vi "Get Path List.vi"(5 "Drivers List":string[](array[string])) -> (4 "APIs Path":path[](array[path]))   [LabVIEW 2021, in "Path Functions.lvlib"]
uses:
  Path Functions.lvlib
  9bdd7397-0e0a-4018-8273-7dcc82681c82.vi
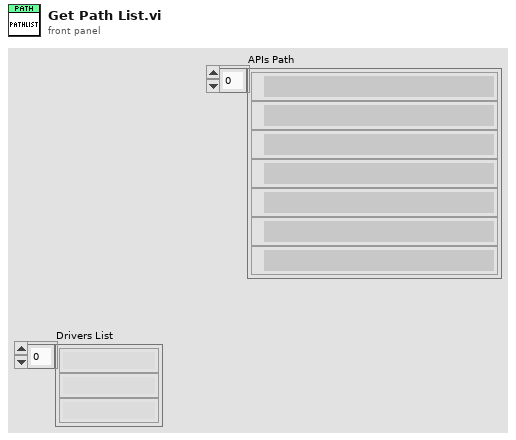
[diagram p1: front panel]
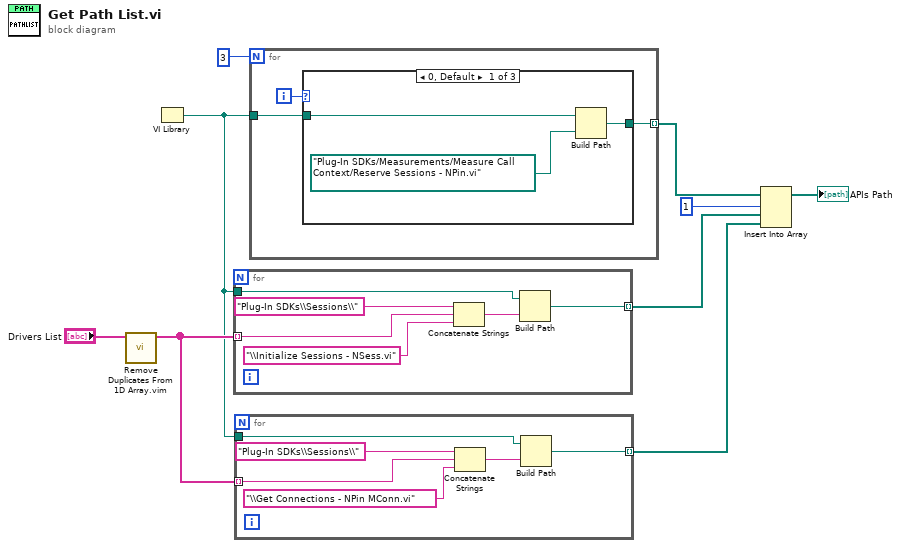
[diagram p0: block diagram]
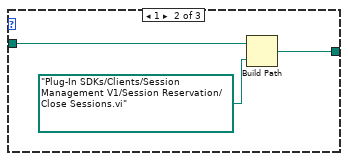
[diagram p2: hidden frame]
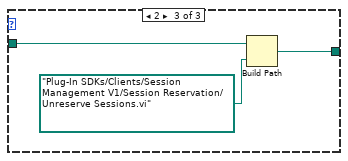
[diagram p3: hidden frame]
diagram:
  n1 = call "Remove Duplicates From 1D Array.vim"("array"="Drivers List") -> ("array with duplicates removed"=w2:string[])  [unwired: 10 in]
  n2 = VI Library() -> (path=w1:path)
  n3 = for {
    tunnel: w2 -> [w13] mode=indexing
    tunnel: w1 -> [w15]
    tunnel: [w10] -> w5 mode=indexing
    n4 = Concatenate Strings("Plug-In SDKs\\Sessions\\" ("string"), w13, "\\Initialize Sessions - NSess.vi" ("string")) -> (w11:string)
    n5 = Build Path(base path=w15, name or relative path=w11) -> (appended path=w10:path)
  }
  n6 = for {
    tunnel: w2 -> [w19] mode=indexing
    tunnel: w1 -> [w21]
    tunnel: [w16] -> w4 mode=indexing
    n7 = Concatenate Strings("Plug-In SDKs\\Sessions\\" ("string"), w19, "\\Get Connections - NPin MConn.vi" ("string")) -> (w17:string)
    n8 = Build Path(base path=w21, name or relative path=w17) -> (appended path=w16:path)
  }
  n9 = for {
    N: 3 -> [_]
    tunnel: w1 -> [w23]
    tunnel: [w22] -> w7 mode=indexing
    i -> [w24]
    n10 = case shown="0, Default" w24 {
      tunnel: w23 -> [w27 w28 w31]
      tunnel: [w25 w29 w32] -> w22
      frame 0, Default {
        n11 = Build Path(base path=w27, name or relative path=path "Plug-In SDKs/Measurements/Measure Call Context/Reserve Sessions - NPin.vi") -> (appended path=w25:path)
      }
      frame 1 {
        n12 = Build Path(base path=w28, name or relative path=path "Plug-In SDKs/Clients/Session Management V1/Session Reservation/Close Sessions.vi") -> (appended path=w29:path)
      }
      frame 2 {
        n13 = Build Path(base path=w31, name or relative path=path "Plug-In SDKs/Clients/Session Management V1/Session Reservation/Unreserve Sessions.vi") -> (appended path=w32:path)
      }
    }
  }
  n14 = Insert Into Array(array=w7, index=1, new element #1=w5, new element #2=w4) -> (→"APIs Path":path[])
